vi "VMI_set_delay_times.vi"(7 "Collection Constant In":T1, 8 "Error In":errorcluster, 10 "Relative Integration Time":dbl=1.0, 11 "Base Integration Time":dbl=30.0) -> (0 "Error Out":errorcluster, 5 "Collection Constant Out":T1)   [LabVIEW 2019]
panel:
  out "x*y":dbl
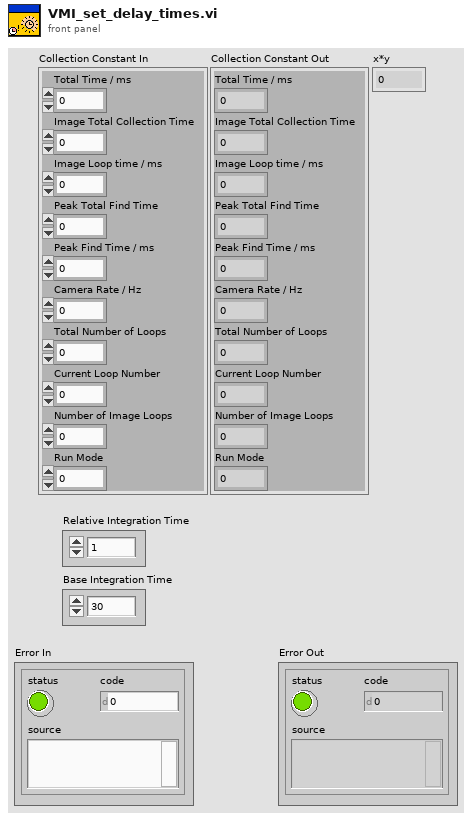
[diagram p1: front panel]
types:
  T1 = cluster{"Total Time / ms":dbl, "Image Total Collection Time":dbl, "Image Loop time / ms":dbl, "Peak Total Find Time":dbl, "Peak Find Time / ms":dbl, "Camera Rate / Hz":dbl, "Total Number of Loops":dbl, "Current Loop Number":dbl, "Number of Image Loops":dbl, "Run Mode":dbl}
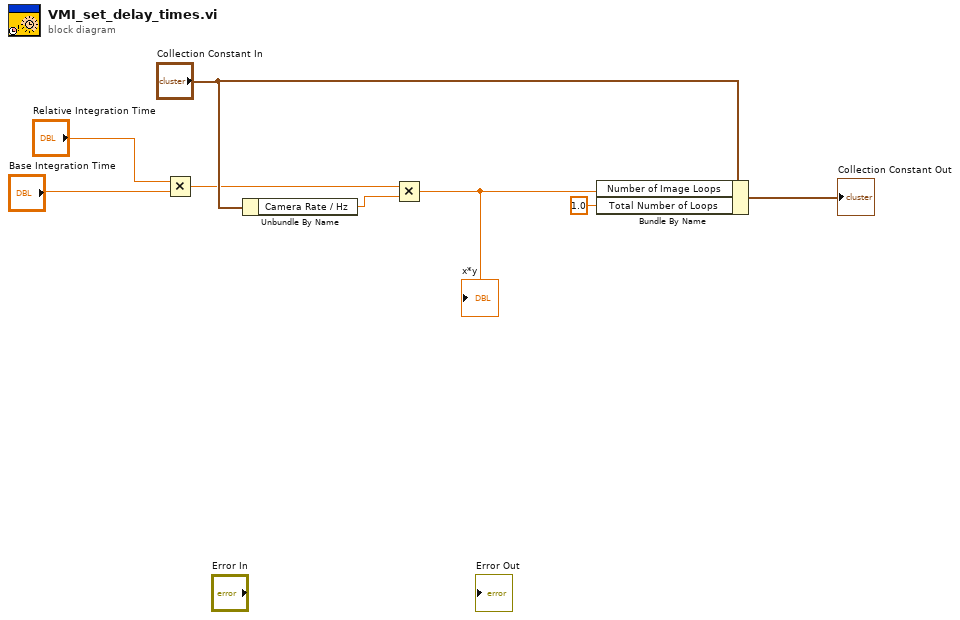
[diagram p0: block diagram]
diagram:
  n1 = Multiply(x="Relative Integration Time", y="Base Integration Time") -> (x*y=w2:dbl)
  n2 = Unbundle By Name("Collection Constant In") -> ("Camera Rate / Hz"=w6:dbl)
  n3 = Multiply(x=w2, y=w6) -> (x*y=w5:dbl)
  "x*y" <- w5
  n4 = Bundle By Name(cluster="Collection Constant In", "Number of Image Loops"=w5, "Total Number of Loops"=1.0) -> (→"Collection Constant Out":T1)
